vi "Write Experiment Folder.vi"(8 "error in (no error)":errorcluster, 10 "Experiment Folder":string, 11 "AFM Control":refnum<class "AFM Control.lvclass">) -> (0 "error out":errorcluster, 3 "AFM Control out":refnum<class "AFM Control.lvclass">)   [LabVIEW 2020, in "AFM Control.lvclass"]
uses:
  AFM Control.lvclass
  AFM Control.lvclass/AFM Control.ctl
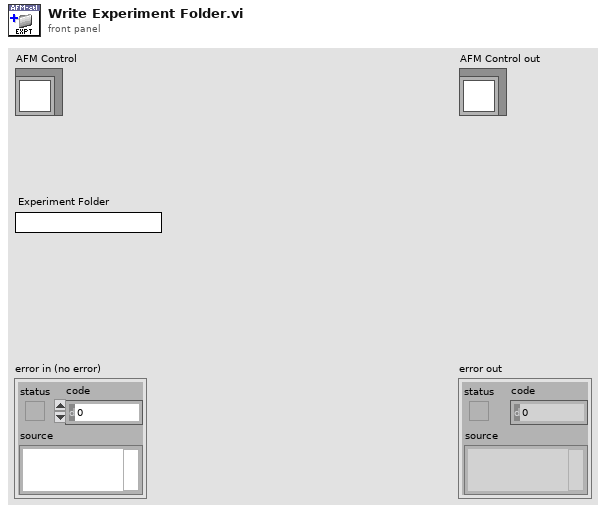
[diagram p1: front panel]
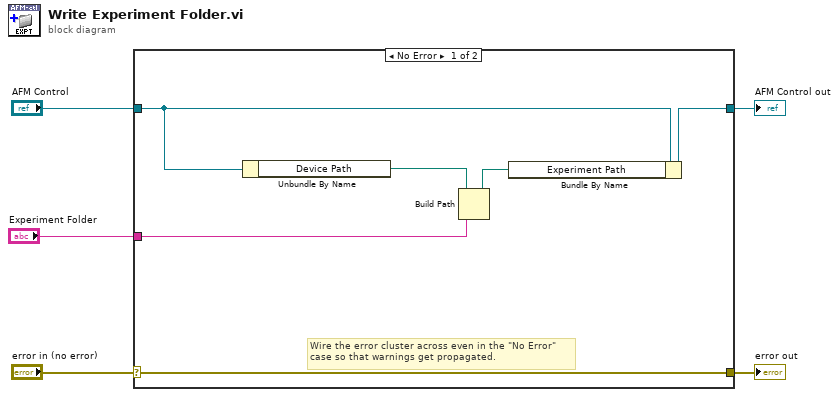
[diagram p0: block diagram]
diagram:
  n1 = case shown="No Error" "error in (no error)" {
    selector: "error in (no error)" -> [w11 w13]
    tunnel: [w11 w13] -> w4
    tunnel: [w6 w12] -> w2
    tunnel: "AFM Control" -> [w7 w12]
    tunnel: "Experiment Folder" -> [w8 _]
    frame No Error {
      # "Wire the error cluster across even in the \"No Error\"\ncase so that warnings get propagated."
      n2 = Unbundle By Name(w7) -> ("Device Path"=w9:path)
      n3 = Build Path(base path=w9, name or relative path=w8) -> (appended path=w10:path)
      n4 = Bundle By Name(cluster=w7, "Experiment Path"=w10) -> (w6:refnum<class "AFM Control.lvclass">)
    }
    frame Error {
    }
  }
  "error out" <- w4
  "AFM Control out" <- w2
